vi "Import Parameters Configuration to New AIM ARINC 429 Custom Device.vi"(7 "Base System Definition File":path=path "Support/Base.nivssdf", 9 "Parameters Configuration File":path=path "Support/Parameters in Scheduled and Dynamic Labels.xml", 10 "Hardware Configuration File":path=path "Support/HW_Rx00_Tx24_Scheduled and Dynamic Labels.xml", 11 "Output System Definition File":path=path "Support/Imported Ballard ARINC 429.nivssdf") -> (3 "Ballard ARINC 429 System Definition":path)   [LabVIEW 2020]
doc: "Overview: Demonstrates using the Ballard ARINC 429 scripting API to configure the custom device by importing a parameters configuration file. \n\nInstructions:\n1. Specify the Parameters Configuration File. This parameters configuration file must be consistent with the schema published on the GitHub repo (https://github.com/ni/niveristand-ballard-arinc429-custom-device/blob/main/Docs/Parameters%20XML%20File/ARINC429_Parameters_XML_Schema.xsd). For successful deployment, the parameters configuration file must also be consistent with the hardware configuration file.\n2. Specify the Hardware Configuration File. The hardware configuration file must be consistent with the schema installed by the Ballard hardware driver at C:\\Program Files (x86)\\Astronics Ballard Technology LabVIEW Driver\\Help\\index.html.\n3. (VeriStand) Optionally, you may open the Ballard ARINC 429 System Definition in VeriStand, configure the PXI Linux RT Target, and deploy the scripted system definition to perform avionics bus communications with Ballard ARINC 429 hardware."
uses:
  AIM ARINC 429 Scripting Examples.lvlib
  <vilib>/addons/VeriStand Custom Device Scripting APIs/Ballard ARINC 429/Custom Device Support/Shared/Initialization Method.ctl
  <vilib>/addons/VeriStand Custom Device Scripting APIs/Ballard ARINC 429/Custom Device Support/Shared/Device Parameters.ctl
  NationalInstruments.VeriStand.SystemDefinitionAPI
panel:
  # "Overview: Demonstrates using the Ballard ARINC 429 scripting API to configure the custom device by importing a parameters configuration file. \n\nInstructions:\n1. Specify the Parameters Configuration File. This parameters configuration file must be consistent with the schema published on the GitHub repo (https://github.com/ni/niveristand-ballard-arinc429-custom-device/blob/main/Docs/Parameters%20XML%20File/ARINC429_Parameters_XML_Schema.xsd). For successful deployment, the parameters configuration file must also be consistent with the hardware configuration file.\n2. Specify the Hardware Configuration File. The hardware configuration file must be consistent with the schema installed by the Ballard hardware driver at C:\\Program Files (x86)\\Astronics Ballard Technology LabVIEW Driver\\Help\\index.html.\n3. (VeriStand) Optionally, you may open the Ballard ARINC 429 System Definition in VeriStand, configure the PXI Linux RT Target, and deploy the scripted system definition to perform avionics bus communications with Ballard ARINC 429 hardware."
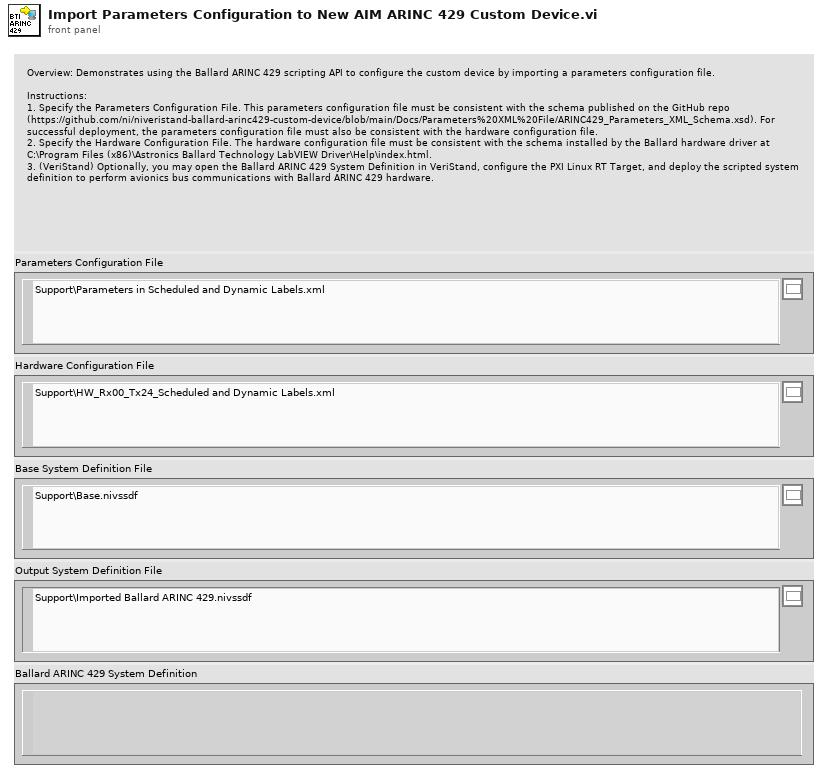
[diagram p1: front panel]
types:
  T1 = typedef "Device Parameters.ctl" = cluster{"initialization method":T2, "card number":i32, "PXI slot number":i32, "core number":i32}
  T2 = typedef "Initialization Method.ctl" = enum16{"PXI Slot Number", "Card Number"}
  T3 = typedef "Custom Device API.lvlib/Custom Device Item Ref.ctl" = u64
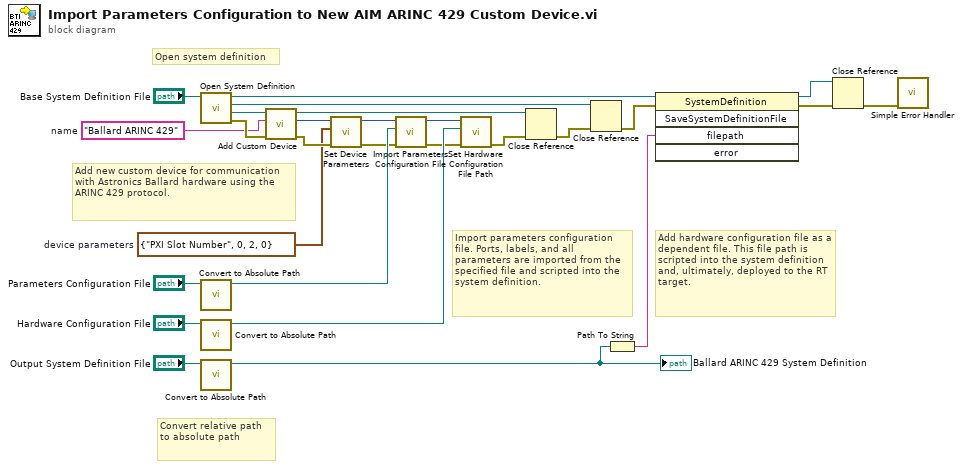
[diagram p0: block diagram]
diagram:
  w1 = T1 {"initialization method"=enum."PXI Slot Number", "card number"=0, "PXI slot number"=2, "core number"=0}  # device parameters
  w15 = "Ballard ARINC 429"  # name
  # "Add hardware configuration file as a dependent file. This file path is scripted into the system definition and, ultimately, deployed to the RT target."
  # "Import parameters configuration file. Ports, labels, and all parameters are imported from the specified file and scripted into the system definition."
  # "Add new custom device for communication with Astronics Ballard hardware using the ARINC 429 protocol."
  # "Convert relative path to absolute path"
  # "Open system definition"
  # "8."
  n1 = call "Open System Definition.vi"("system definition file"="Base System Definition File") -> ("error out"=w16:errorcluster, "target"=w17:refnum<k24>, "root"=w19:refnum<k24>, "system definition"=w20:refnum<k24>)  [unwired: 7 in]
  n2 = call "Convert to Absolute Path.vi"("system definition file"="Parameters Configuration File") -> ("absolute path"=w13:path)  [unwired: 10 in]
  n3 = call "Convert to Absolute Path.vi"("system definition file"="Hardware Configuration File") -> ("absolute path"=w11:path)  [unwired: 10 in]
  n4 = call "Convert to Absolute Path.vi"("system definition file"="Output System Definition File") -> ("absolute path"=w6:path)  [unwired: 10 in]
  "Ballard ARINC 429 System Definition" <- w6
  n5 = call <vilib>:"Add Custom Device.vi"("error in"=w16, "name"=w15, "target in"=w17) -> ("error out"=w3:errorcluster, "Ballard ARINC 429 custom device"=w5:T3, "target out"=w7:refnum<k24>)  [unwired: 6 in]
  n6 = call <vilib>:"Set Device Parameters.vi"("error in"=w3, "device parameters"=w1, "Ballard ARINC 429 custom device in"=w5) -> ("error out"=w2:errorcluster, "Ballard ARINC 429 custom device out"=w4:T3)  [unwired: 7 in]
  n7 = call <vilib>:"Import Parameters Configuration File.vi"("error in"=w2, "parameters configuration file path"=w13, "Ballard ARINC 429 custom device in"=w4) -> ("error out"=w9:errorcluster, "Ballard ARINC 429 custom device out"=w10:T3)  [unwired: 7 in]
  n8 = call <vilib>:"Set Hardware Configuration File Path.vi"("error in"=w9, "hardware configuration file path"=w11, "Ballard ARINC 429 custom device in"=w10) -> ("error out"=w8:errorcluster)  [unwired: 7 in, 1 out]
  n9 = Close Reference(reference=w7, error in (no error)=w8) -> (error out=w18:errorcluster)
  n10 = Close Reference(reference=w19, error in (no error)=w18) -> (error out=w23:errorcluster)
  n11 = Path To String(path=w6) -> (string=w26:string)
  n12 = invoke class="SystemDefinition" method="SaveSystemDefinitionFile"(reference=w20, error in=w23, "filepath"=w26) -> (reference out=w24:refnum<k24>, error out=w25:errorcluster)  [unwired: 2 in, 3 out]
  n13 = Close Reference(reference=w24, error in (no error)=w25) -> (error out=w22:errorcluster)
  n14 = call <vilib>:"Simple Error Handler.vi"("error in (no error)"=w22) -> ()  [unwired: 1 in, 8 out]
